vi "oax_gsData Logger (DAQmx).vi"() -> ()   [LabVIEW 2017]
uses:
  <vilib>/addons/Sound and Vibration/Order Analysis/Example Support/sub VIs/OAXML_DSA DAQ Config.ctl
  <vilib>/addons/_NISVFA/_Shared subVIs/Controls/svc_Engineering Units Text Ring.ctl
  <vilib>/DAQmx/read.llb/DAQmx Read (Analog 2D DBL NChan NSamp).vi
  <vilib>/DAQmx/miscellaneous.llb/DAQmx Fill In Error Info.vi
  <vilib>/DAQmx/configure/timing.llb/DAQmx Timing (Sample Clock).vi
panel:
  in  "stop":bool
  out "Waveform Chart":sgl[][](graph)
  out "coefficients":dbl[](array[numeric]) format="%.2f"
  out "tacho channel index":i32
  in  "DAQ Configuration":bool
  out "TF Plot":dbl[][](graph) caption="Time-Frequency Plot"
  out "Spectrum":cluster{"x[i]":dbl[], "y[i]":dbl[]}(graph)
  out "# of points\nsaved":i32
  out "# of points\nsampled":i32
  in  "Display Signal":u16(ring) items=["CH1", "CH2", "CH3"]
  in  "Window Type":u16(ring)=3 items=["Rectangular", "Blackman", "Hamming", "Hanning", "Gaussian"]
  in  "Window Length":u16(ring)=2 items=["256", "512", "1024", "2048", "4096"]
  in  "Save":bool
  in  "Start DAQ":bool
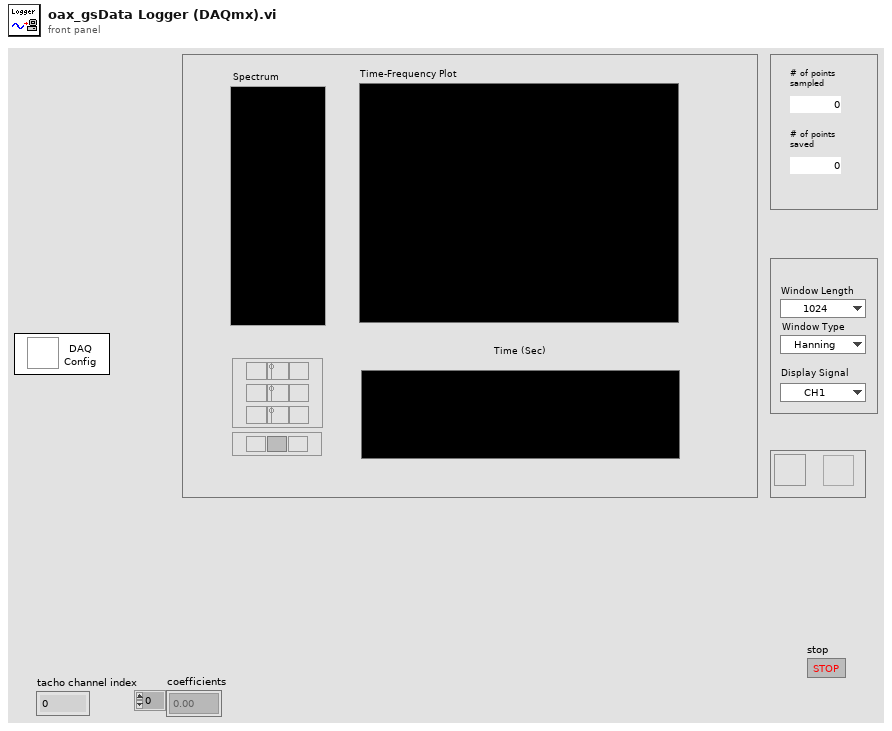
[diagram p1: front panel]
types:
  T1 = typedef "OAXML_DSA DAQ Config.ctl" = cluster{"name":string, "channel":tag, "coupling":u16, "dB reference":sgl, "sensor sensitivity (mV/EU)":dbl, "engineering units":T2, "IEPE":u16, "custom label":string, "pregain":sgl}[]
  T2 = typedef "svc_Engineering Units Text Ring.ctl" = u16
  T3 = cluster{"tachometer channel":tag, "sample rate [samples/s]":dbl, "Max Value":dbl, "Min Value":dbl, "Path":path}
  T4 = typedef "LVRangeTypeDef.ctl" = cluster{"Minimum":dbl, "Maximum":dbl, "Increment":dbl, "Minor Increment":dbl, "Start":dbl}
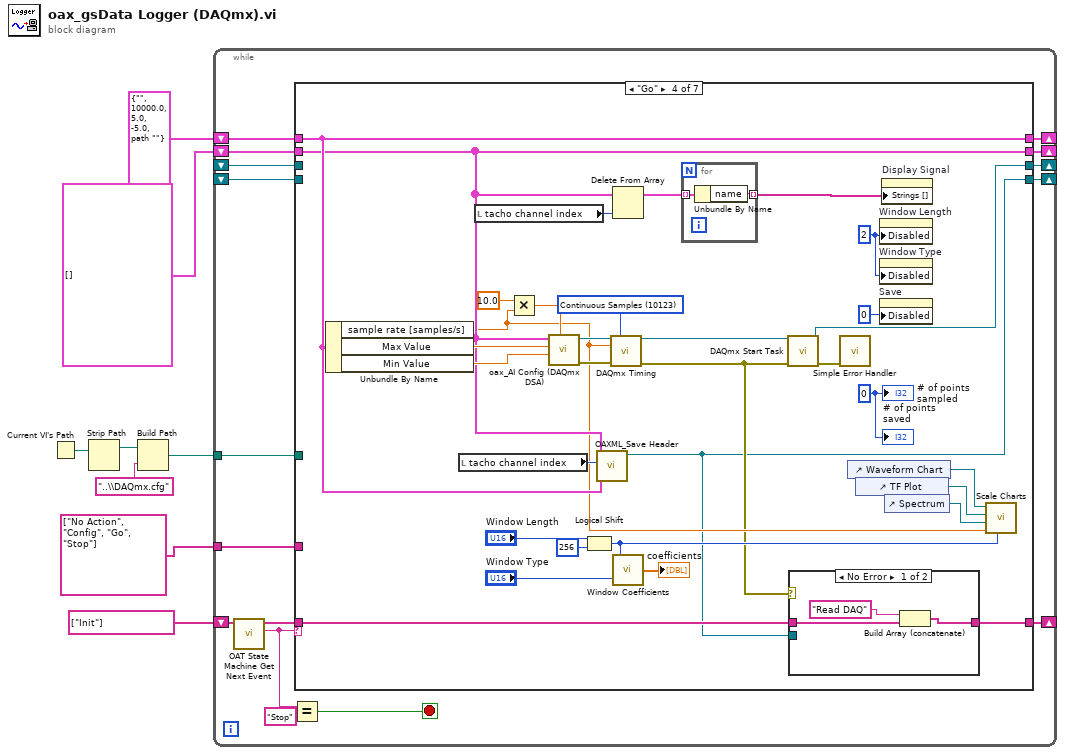
[diagram p0: block diagram]
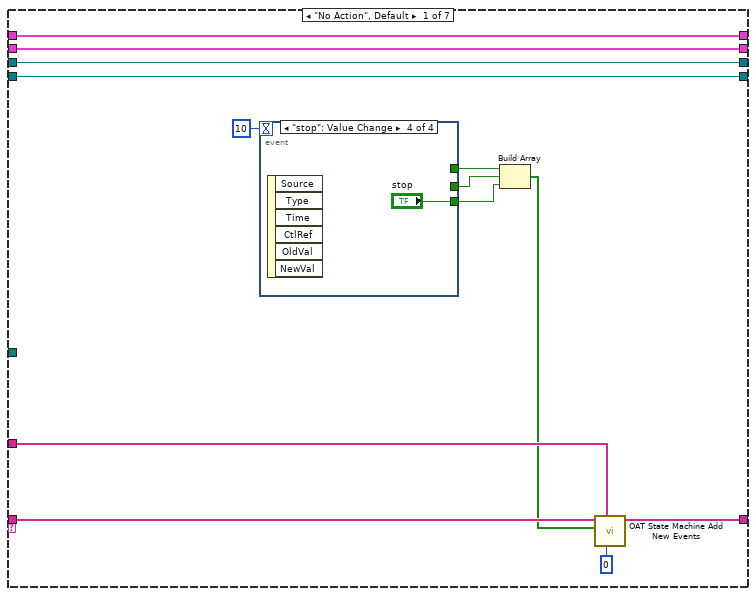
[diagram p2: hidden frame]
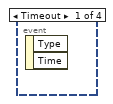
[diagram p3: hidden frame]
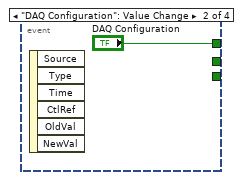
[diagram p4: hidden frame]
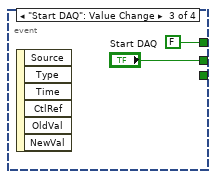
[diagram p5: hidden frame]
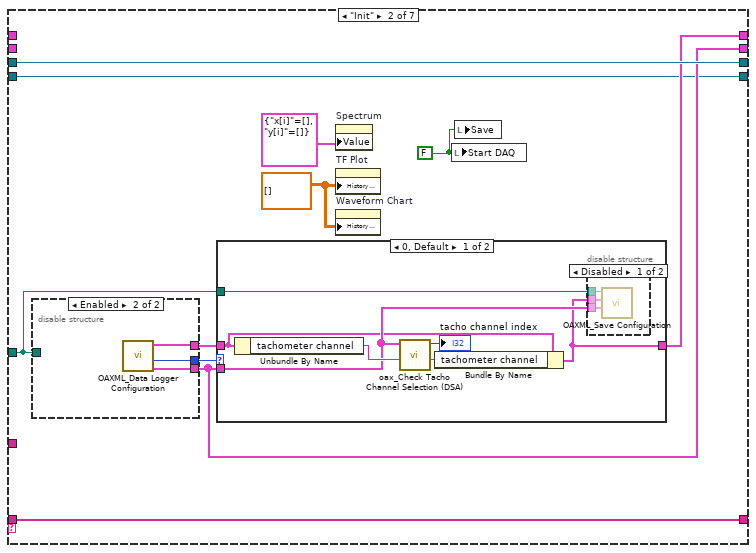
[diagram p6: hidden frame]
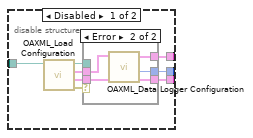
[diagram p7: hidden frame]
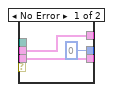
[diagram p8: hidden frame]
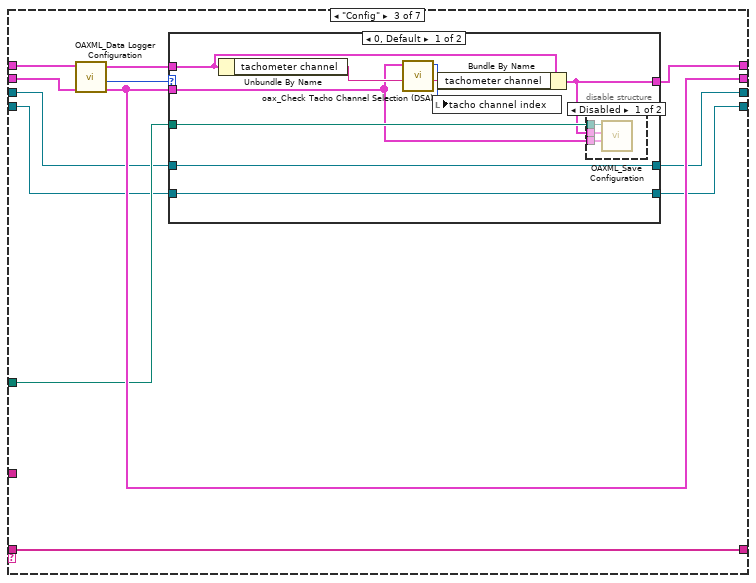
[diagram p11: hidden frame]
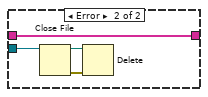
[diagram p14: hidden frame]
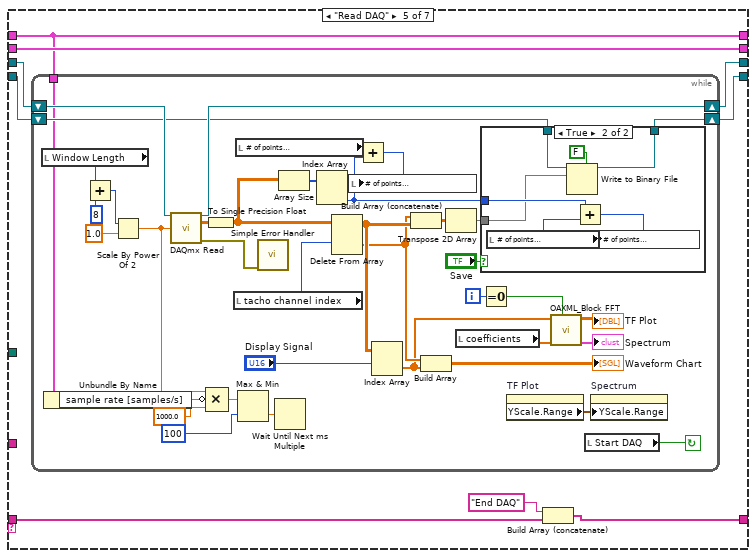
[diagram p15: hidden frame]
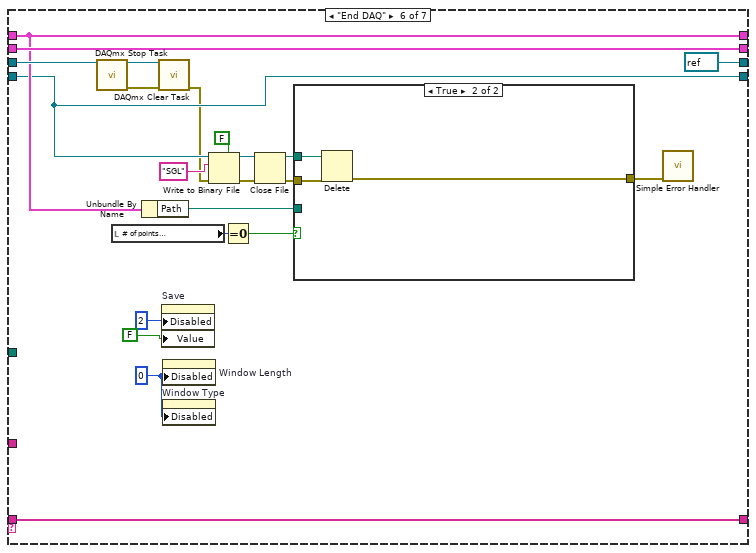
[diagram p17: hidden frame]
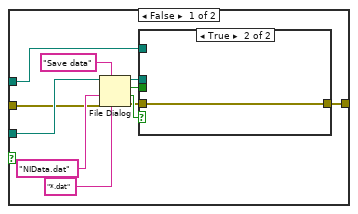
[diagram p18: hidden frame]
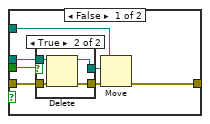
[diagram p19: hidden frame]
diagram:
  n1 = Current VI's Path() -> (path=w5:path)
  n2 = Strip Path(path=w5) -> (stripped path=w7:path)  [unwired: 1 out]
  n3 = Build Path(base path=w7, name or relative path="..\\DAQmx.cfg") -> (appended path=w4:path)
  n4 = while {
    shift-right: [w16] -> _
    shift-left: string[] ["Init"] -> [w24]
    tunnel: w4 -> [w19]
    shift-right: [w17] -> _
    shift-left: T1 [] ("DAQ Config in") -> [w14]
    shift-right: [w18] -> _
    shift-left: T3 {"tachometer channel"="", "sample rate [samples/s]"=10000.0, "Max Value"=5.0, "Min Value"=-5.0, "Path"=path ""} ("Param in") -> [w15]
    tunnel: string[] ["No Action", "Config", "Go", "Stop"] -> [w13]
    shift-right: [w12] -> _
    shift-left: _ -> [w11]
    shift-right: [w10] -> _
    shift-left: _ -> [w9]
    stop <- w22 stop-if-true
    n5 = call <vilib>:"OAT State Machine Get Next Event.vi"("event queue in"=w24) -> ("next event"=w21:string, "event queue out"=w20:string[])  [unwired: 5 in]
    n6 = Equal?(x=w21, y="Stop") -> (x = y?=w22:bool)
    n7 = case shown="\"Go\"" w21 {
      tunnel: w20 -> [w35 w52 w91 w132 w154 w214 w256]
      tunnel: w19 -> [_ w49 w87 _ _ _ _]
      tunnel: [w37 w47 w90 w133 w151 w220 w260] -> w18
      tunnel: [w36 w48 w89 w128 w159 w227 w259] -> w17
      tunnel: [w33 w52 w91 w131 w153 w214 w256] -> w16
      tunnel: w15 -> [w37 _ w93 w133 w151 w220 w260]
      tunnel: w14 -> [w36 _ w92 w128 w159 w227 w259]
      tunnel: w13 -> [w34 _ _ _ _ _ _]
      tunnel: [w27 w51 w86 w135 w157 refnum<k21> refnum ("task out") w258] -> w12
      tunnel: w11 -> [w27 w51 w85 _ w158 w226 w258]
      tunnel: [w26 w45 w83 w110 w155 w217 w257] -> w10
      tunnel: w9 -> [w26 w45 w84 _ w156 w217 w257]
      frame "No Action", Default {
        n8 = event shown="[3] \"stop\": Value Change" {
          selector: _ -> [_ _ _ _]
          dyn-events: _ -> [_ _ _ _]
          timeout: 10 -> [_ _ _ _]
          tunnel: [_ "DAQ Configuration" FALSE ("DAQ Configuration") _] -> w29
          tunnel: [_ _ "Start DAQ" _] -> w28
          tunnel: [_ _ _ "stop"] -> w25
          event Timeout {
            n9 = event-data() -> ()  [unwired: 1 in, 2 out]
          }
          event "DAQ Configuration": Value Change {
            n10 = event-data() -> ()  [unwired: 1 in, 6 out]
          }
          event "Start DAQ": Value Change {
            n11 = event-data() -> ()  [unwired: 1 in, 6 out]
          }
          event "stop": Value Change {
            n12 = event-data() -> ()  [unwired: 1 in, 6 out]
          }
        }
        n13 = Build Array(w29, w28, w25) -> (w32:bool[])
        n14 = call <vilib>:"OAT State Machine Add New Events.vi"("ms timeout (200)"=0, "Event Names"=w34, "New Events"=w32, "Event Queue In"=w35) -> ("Event Queue Out"=w33:string[])  [unwired: 7 in]
      }
      frame "Init" {
        w42 = dbl[][] [] ("History Data")
        w44 = FALSE ("Start DAQ")
        n15 = disable-structure shown="Enabled" {
          disable-tunnel: [w56 w69] -> w50
          disable-tunnel: w49 -> [w55 _]
          disable-tunnel: [w54 w71] -> w48
          disable-tunnel: [w53 w70] -> w46
          frame Disabled {
            n16 = call <vilib>:"OAXML_Load Configuration.vi"("config file"=w55) -> ("error out"=w60:errorcluster, "DAQ Configuration out"=w59:T1, "param out"=w58:T3, "config file out"=w57:path)  [unwired: 7 in]
            n17 = case shown="Error" w60 {
              tunnel: w59 -> [w62 w67]
              tunnel: w58 -> [w63 w68]
              tunnel: w57 -> [_ _]
              tunnel: [w63 w65] -> w56
              tunnel: [w62 w66] -> w54
              tunnel: [u16 0 ("result") w64] -> w53
              frame No Error {
              }
              frame Error {
                n18 = call <vilib>:"OAXML_Data Logger Configuration.vi"("DAQ Config in"=w67, "Param in"=w68) -> ("DAQ Config out"=w66:T1, "result"=w64:u16, "Param out"=w65:T3)  [unwired: 7 in]
              }
            }
          }
          frame Enabled {
            n19 = call <vilib>:"OAXML_Data Logger Configuration.vi"() -> ("DAQ Config out"=w71:T1, "result"=w70:u16, "Param out"=w69:T3)  [unwired: 9 in]
          }
        }
        n20 = case shown="0, Default" w46 {
          tunnel: w50 -> [w74 w82]
          tunnel: [w73 w82] -> w47
          tunnel: w48 -> [w75 _]
          tunnel: w49 -> [w76 _]
          frame 0, Default {
            n21 = Unbundle By Name(w74) -> ("tachometer channel"=w78:tag)
            n22 = call <vilib>:"oax_Check Tacho Channel Selection (DSA).vi"("tachometer channel"=w78, "DAQ Config"=w75) -> ("tachometer channel selected"=w77:tag, "tacho channel index"=→"tacho channel index":i32)  [unwired: 6 in, 2 out]
            n23 = Bundle By Name(cluster=w74, "tachometer channel"=w77) -> (w73:T3)
            n24 = disable-structure shown="Disabled" {
              disable-tunnel: w76 -> [w81 _]
              disable-tunnel: w75 -> [w80 _]
              disable-tunnel: w73 -> [w79 _]
              frame Disabled {
                n25 = call <vilib>:"OAXML_Save Configuration.vi"("DAQ Config in"=w80, "Param in"=w79, "config file"=w81) -> ()  [unwired: 7 in, 2 out]
              }
              frame Enabled {
              }
            }
          }
          frame 1 {
          }
        }
        n26 = property on="Spectrum" class="XYGraph (strict)"("Value"=cluster{"x[i]":dbl[], "y[i]":dbl[]} {"x[i]"=[], "y[i]"=[]} ("Spectrum")) -> ()  [unwired: 2 in, 2 out]
        n27 = property on="TF Plot" class="IntChart (strict)"("History Data"=w42) -> ()  [unwired: 2 in, 2 out]
        n28 = property on="Waveform Chart" class="WFChart (strict)"("History Data"=w42) -> ()  [unwired: 2 in, 2 out]
        n29 = local write "Start DAQ"(w44) -> ()
        n30 = local write "Save"(w44) -> ()
      }
      frame "Config" {
        n31 = call <vilib>:"OAXML_Data Logger Configuration.vi"("DAQ Config in"=w92, "Param in"=w93) -> ("DAQ Config out"=w89:T1, "result"=w88:u16, "Param out"=w94:T3)  [unwired: 7 in]
        n32 = case shown="0, Default" w88 {
          tunnel: w94 -> [w103 w109]
          tunnel: [w99 w109] -> w90
          tunnel: w89 -> [w98 _]
          tunnel: w87 -> [w100 _]
          tunnel: [w97 w108] -> w86
          tunnel: w85 -> [w97 w108]
          tunnel: [w95 w107] -> w83
          tunnel: w84 -> [w95 w107]
          frame 0, Default {
            n33 = Unbundle By Name(w103) -> ("tachometer channel"=w102:tag)
            n34 = call <vilib>:"oax_Check Tacho Channel Selection (DSA).vi"("tachometer channel"=w102, "DAQ Config"=w98) -> ("tachometer channel selected"=w101:tag, "tacho channel index"=w96:i32)  [unwired: 6 in, 2 out]
            n35 = local write "tacho channel index"(w96) -> ()
            n36 = Bundle By Name(cluster=w103, "tachometer channel"=w101) -> (w99:T3)
            n37 = disable-structure shown="Disabled" {
              disable-tunnel: w100 -> [w106 _]
              disable-tunnel: w99 -> [w105 _]
              disable-tunnel: w98 -> [w104 _]
              frame Disabled {
                n38 = call <vilib>:"OAXML_Save Configuration.vi"("DAQ Config in"=w104, "Param in"=w105, "config file"=w106) -> ()  [unwired: 7 in, 2 out]
              }
              frame Enabled {
              }
            }
          }
          frame 1 {
          }
        }
      }
      frame "Go" {
        w116 = u8 2 ("Disabled")
        w130 = 0 ("# of points\nsampled")
        w140 = 10123 items=["Finite Samples"=10178, "Continuous Samples"=10123, "Hardware Timed Single Point"=12522] ("sample mode")
        n39 = Unbundle By Name(w133) -> ("sample rate [samples/s]"=w112:dbl, "Max Value"=w141:dbl, "Min Value"=w137:dbl)
        n40 = local read "tacho channel index"() -> (w134:i32)
        n41 = local read "tacho channel index"() -> (w127:i32)
        n42 = Multiply(x=10.0 ("y"), y=w112) -> (x*y=w114:dbl)
        n43 = call <vilib>:"oax_AI Config (DAQmx DSA).vi"("buffer size"=w114, "min value"=w137, "max value"=w141, "DAQ Config"=w128) -> ("error out"=w138:errorcluster, "task out"=w139:refnum<k21>)  [unwired: 6 in]
        n44 = Logical Shift(y="Window Length", x=256 ("Min of WinLen")) -> (x << y=w120:i32)
        n45 = call <vilib>:"OAXML_Save Header.vi"("Param in"=w133, "tacho channel index"=w134, "DAQ Config"=w128) -> ("file refnum"=w110:refnum<file>)  [unwired: 8 in]
        n46 = call-poly <vilib>:"DAQmx Timing.vi"("task/channels in"=w139, "sample mode"=w140, "rate"=w112, "error in"=w138) -> ("task out"=w136:refnum<k21>, "error out"=w111:errorcluster)  [unwired: 10 in]
        n47 = Delete From Array(array=w128, index=w127) -> (array with subset deleted=w126:T1)  [unwired: 1 in, 1 out]
        n48 = call <vilib>:"Window Coefficients.vi"("window type"="Window Type", "window length"=w120) -> ("coefficients"=→"coefficients":dbl[])
        n49 = for {
          tunnel: w126 -> [w150] mode=indexing
          tunnel: [w149] -> w125 mode=indexing
          n50 = Unbundle By Name(w150) -> ("name"=w149:string)
        }
        n51 = call <vilib>:"DAQmx Start Task.vi"("task/channels in"=w136, "error in"=w111) -> ("task out"=w135:refnum<k21>, "error out"=w115:errorcluster)  [unwired: 12 in]
        n52 = case shown="No Error" w111 {
          tunnel: w132 -> [w144 w148]
          tunnel: [w143 w148] -> w131
          tunnel: w110 -> [_ w147]
          frame No Error {
            n53 = Build Array (concatenate)("Read DAQ", w144) -> (w143:string[])
          }
          frame Error {
            n54 = Close File(refnum=w147) -> (path=w145:path, error out=w146:errorcluster)  [unwired: 1 in]
            n55 = Delete(path (use dialog)=w145, error in=w146) -> ()  [unwired: 3 in, 3 out]
          }
        }
        n56 = call <vilib>:"Simple Error Handler.vi"("error in (no error)"=w115) -> ()  [unwired: 4 in, 5 out]
        n57 = control-ref of="Waveform Chart"() -> (w117:refnum<vi>)
        n58 = control-ref of="TF Plot"() -> (w119:refnum<vi>)
        n59 = property on="Window Length" class="Ring (strict)"("Disabled"=w116) -> ()  [unwired: 2 in, 2 out]
        n60 = property on="Window Type" class="Ring (strict)"("Disabled"=w116) -> ()  [unwired: 2 in, 2 out]
        n61 = property on="Save" class="Bool (strict)"("Disabled"=u8 0) -> ()  [unwired: 2 in, 2 out]
        n62 = property on="Display Signal" class="Ring (strict)"("Strings []"=w125) -> ()  [unwired: 2 in, 2 out]
        n63 = control-ref of="Spectrum"() -> (w118:refnum<vi>)
        n64 = call <vilib>:"Scale Charts.vi"("window length"=w120, "sample rate"=w112, "XY Grahp"=w118, "IntesityChart"=w119, "Waveform Chart"=w117) -> ()  [unwired: 6 in]
        "# of points\nsampled" <- w130
        "# of points\nsaved" <- w130
      }
      frame "Read DAQ" {
        n65 = while {
          shift-right: [w196] -> w157
          shift-left: w158 -> [w197]
          shift-right: [w189] -> w155
          shift-left: w156 -> [w190]
          tunnel: w151 -> [w168]
          i -> [w178]
          stop <- w188 continue-if-true
          n66 = local read "Window Length"() -> (w169:u16)
          n67 = Unbundle By Name(w168) -> ("sample rate [samples/s]"=w166:dbl)
          n68 = Add(x=w169, y=u16 8) -> (x+y=w172:u16)
          n69 = Scale By Power Of 2(n=w172, x=1.0) -> (x*2^n=w165:dbl)
          n70 = call-poly <vilib>:"DAQmx Read.vi"("task/channels in"=w197, "number of samples per channel"=w165) -> ("task out"=w196:refnum<k21>, "data"=w187:dbl[][], "error out"=w160:errorcluster)  [unwired: 11 in]
          n71 = To Single Precision Float(number=w187) -> (single precision float=w186:sgl[][])
          n72 = Compound Arithmetic op=MULTIPLY(w165, invert w166, 1000.0 ("value")) -> (w164:dbl)
          n73 = local read "tacho channel index"() -> (w195:i32)
          n74 = local read "# of points\nsampled"() -> (w192:i32)
          n75 = Max & Min(x=w164, y=u32 100 ("millisecond multiple")) -> (min(x,y)=w162:dbl)  [unwired: 1 out]
          n76 = call <vilib>:"Simple Error Handler.vi"("error in (no error)"=w160) -> ()  [unwired: 4 in, 5 out]
          n77 = Wait Until Next ms Multiple(millisecond multiple=w162) -> ()  [unwired: 1 out]
          n78 = Array Size(array=w186) -> (size(s)=w193:i32[])
          n79 = Index Array(array=w193) -> (element #2=w177:i32)  [unwired: 2 in, 1 out]
          n80 = Delete From Array(array=w186, index (row)=w195) -> (deleted portion=w179:sgl[], array with subset deleted=w183:sgl[][])  [unwired: 2 in]
          n81 = Add(x=w192, y=w177) -> (x+y=w191:i32)
          n82 = local write "# of points\nsampled"(w191) -> ()
          n83 = Index Array(array=w183, index (row)="Display Signal") -> (element=w161:sgl[])  [unwired: 1 in]
          n84 = Build Array (concatenate)(w179, w183) -> (w185:sgl[][])
          n85 = Build Array(w179, w161) -> (→"Waveform Chart":sgl[][])
          n86 = Transpose 2D Array(2D array=w185) -> (transposed array=w184:sgl[][])
          n87 = local read "coefficients"() -> (w175:dbl[])
          n88 = case shown="True" "Save" {
            tunnel: w184 -> [_ w200]
            tunnel: w177 -> [_ w204]
            tunnel: w190 -> [w198 w201]
            tunnel: [w198 w199] -> w189
            frame False {
            }
            frame True {
              n89 = local read "# of points\nsaved"() -> (w203:i32)
              n90 = Write to Binary File(file (use dialog)=w201, data=w200, 5:FALSE ("prepend array or string size? (T)")) -> (refnum out=w199:refnum<file>)  [unwired: 3 in, 2 out]
              n91 = Add(x=w204, y=w203) -> (x+y=w205:i32)
              n92 = local write "# of points\nsaved"(w205) -> ()
            }
          }
          n93 = Equal To 0?(x=w178) -> (x = 0?=w176:bool)
          n94 = property on="TF Plot" class="IntChart (strict)"() -> ("YScale.Range"=w180:T4)  [unwired: 2 in, 2 out]
          n95 = call <vilib>:"OAXML_Block FFT.vi"("Reset(F)"=w176, "window coefficients"=w175, "X"=w161) -> ("Last Spectrum"=→"Spectrum":cluster{"x[i]":dbl[], "y[i]":dbl[]}, "Block FFT Spectrum"=→"TF Plot":dbl[][])  [unwired: 7 in]
          n96 = local read "Start DAQ"() -> (w188:bool)
          n97 = property on="Spectrum" class="XYGraph (strict)"("YScale.Range"=w180) -> ()  [unwired: 2 in, 2 out]
        }
        n98 = Build Array (concatenate)("End DAQ" ("y"), w154) -> (w153:string[])
      }
      frame "End DAQ" {
        w211 = u8 0 ("Disabled")
        n99 = call <vilib>:"DAQmx Stop Task.vi"("task/channels in"=w226) -> ("task out"=w210:refnum<k21>, "error out"=w209:errorcluster)  [unwired: 13 in]
        n100 = local read "# of points\nsaved"() -> (w218:i32)
        n101 = Unbundle By Name(w220) -> ("Path"=w219:path)
        n102 = call <vilib>:"DAQmx Clear Task.vi"("task in"=w210, "error in"=w209) -> ("error out"=w208:errorcluster)  [unwired: 13 in]
        n103 = property on="Save" class="Bool (strict)"("Disabled"=u8 2, "Value"=FALSE ("Save")) -> ()  [unwired: 2 in, 2 out]
        n104 = property on="Window Length" class="Ring (strict)"("Disabled"=w211) -> ()  [unwired: 2 in, 2 out]
        n105 = property on="Window Type" class="Ring (strict)"("Disabled"=w211) -> ()  [unwired: 2 in, 2 out]
        n106 = Write to Binary File(file (use dialog)=w217, data="SGL", error in=w208, 5:FALSE ("prepend array or string size? (T)")) -> (refnum out=w223:refnum<file>, error out=w216:errorcluster)  [unwired: 2 in, 1 out]
        n107 = Equal To 0?(x=w218) -> (x = 0?=w221:bool)
        n108 = Close File(refnum=w223, error in=w216) -> (path=w222:path, error out=w215:errorcluster)
        n109 = case shown="True" w221 {
          tunnel: w222 -> [w235 w255]
          tunnel: w219 -> [w234 _]
          tunnel: w215 -> [w230 w254]
          tunnel: [w228 w253] -> w206
          frame False {
            n110 = File Dialog(6:"*.dat", 7:"Save data" ("prompt"), 8:w230, 9:"NIData.dat" ("default name"), 11:w234) -> (0:w229:errorcluster, 1:w233:bool, 2:w232:bool, 3:w236:path)  [unwired: 2 in]
            n111 = case shown="True" w233 {
              tunnel: w236 -> [w245 _]
              tunnel: w235 -> [w244 _]
              tunnel: w232 -> [w240 _]
              tunnel: w229 -> [w242 w252]
              tunnel: [w239 w252] -> w228
              frame False {
                n112 = case shown="True" w240 {
                  tunnel: w245 -> [w247 w251]
                  tunnel: [w247 w250] -> w243
                  tunnel: w242 -> [w246 w249]
                  tunnel: [w246 w248] -> w241
                  frame False {
                  }
                  frame True {
                    n113 = Delete(path (use dialog)=w251, error in=w249) -> (deleted path=w250:path, error out=w248:errorcluster)  [unwired: 3 in, 1 out]
                  }
                }
                n114 = Move(source path=w244, error in=w241, 10:w243) -> (error out=w239:errorcluster)  [unwired: 2 in, 2 out]
              }
              frame True {
              }
            }
          }
          frame True {
            n115 = Delete(path (use dialog)=w255, error in=w254) -> (error out=w253:errorcluster)  [unwired: 3 in, 2 out]
          }
        }
        n116 = call <vilib>:"Simple Error Handler.vi"("error in (no error)"=w206) -> ()  [unwired: 4 in, 5 out]
      }
      frame "Stop" {
      }
    }
  }
